vi "Test TEMPLATE.vi"(8 "error in (no error)":errorcluster) -> (0 "error out":errorcluster)   [LabVIEW 2020, in "TEST JKI State Machine API.lvlib"]
uses:
  TEST JKI State Machine API.lvlib
  source/JKI SM/JKI SM.lvclass
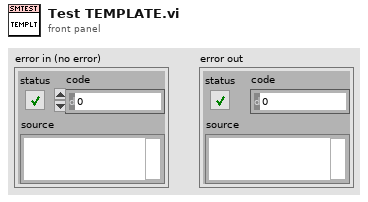
[diagram p1: front panel]
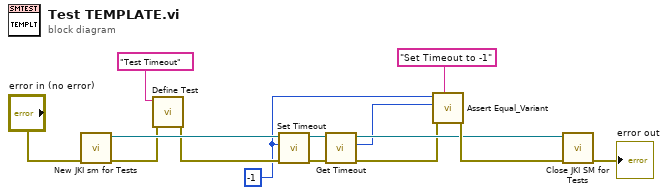
[diagram p0: block diagram]
diagram:
  w4 = -1 ("Timeout (ms)")
  n1 = call "New JKI sm for Tests.vi"("error in (no error)"="error in (no error)") -> ("error out"=w13:errorcluster, "JKI SM out"=w14:refnum<class "JKI SM.lvclass">)  [unwired: 9 in]
  n2 = call <vilib>:"Define Test.vi"("error in (no error)"=w13, "Label (VI Title)"="Test Timeout") -> ("error out"=w11:errorcluster)  [unwired: 8 in, 1 out]
  n3 = call "Set Timeout.vi"("error in (no error)"=w11, "Timeout (ms)"=w4, "JKI SM in"=w14) -> ("error out"=w2:errorcluster, "JKI SM out"=w3:refnum<class "JKI SM.lvclass">)  [unwired: 7 in]
  n4 = call "Get Timeout.vi"("error in (no error)"=w2, "JKI SM in"=w3) -> ("error out"=w7:errorcluster, "Timeout (ms)"=w5:i32, "JKI SM out"=w8:refnum<class "JKI SM.lvclass">)  [unwired: 7 in]
  n5 = call <vilib>:"Assert Equal_Variant.vi"("Label"="Set Timeout to -1", "error in (no error)"=w7, "Y"=w5, "X"=w4) -> ("error out"=w9:errorcluster)  [unwired: 7 in]
  n6 = call "Close JKI SM for Tests.vi"("error in (no error)"=w9, "JKI SM in"=w8) -> ("error out"=→"error out":errorcluster)  [unwired: 9 in]
